vi "FactorialsFinder.vi"() -> ()   [LabVIEW 2019]
panel:
  out "factorial indicator":dbl
  in  "Number for factorials":dbl
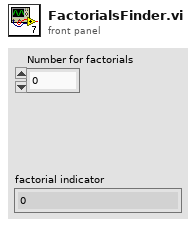
[diagram p1: front panel]
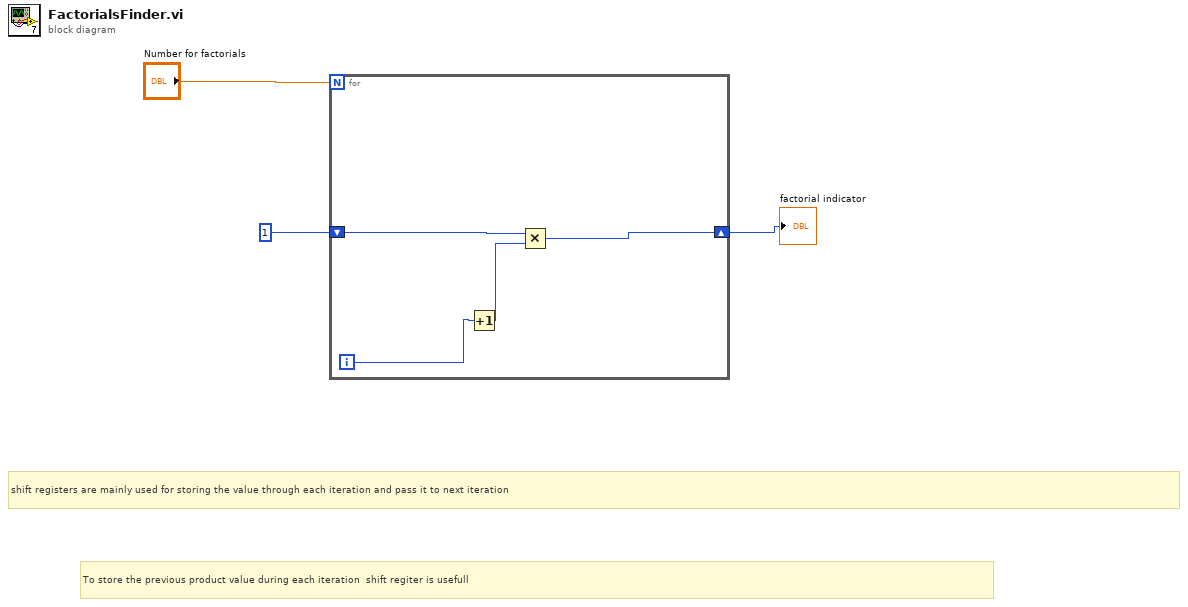
[diagram p0: block diagram]
diagram:
  # "To store the previous product value during each iteration  shift regiter is usefull"
  # "shift registers are mainly used for storing the value through each iteration and pass it to next iteration"
  n1 = for {
    N: "Number for factorials" -> [_]
    shift-right: [w4] -> w1
    shift-left: 1 -> [w7]
    i -> [w6]
    n2 = Increment(x=w6) -> (x+1=w5:i32)
    n3 = Multiply(x=w7, y=w5) -> (x*y=w4:i32)
  }
  "factorial indicator" <- w1
